vi "FiberWLC_CalcState.vi"(5 "Distribution of states":i32[][](array[numeric]), 7 "Li (bp)":dbl[](array[numeric]), 8 "Gi (kT)":dbl[](array[numeric]), 9 "L handles (bp)":dbl) -> (1 "L free (bp)":dbl[](array[numeric]), 2 "ni*Gi (kT)":dbl[](array[numeric]), 3 "n0":i32[](array[numeric]))   [LabVIEW 2018]
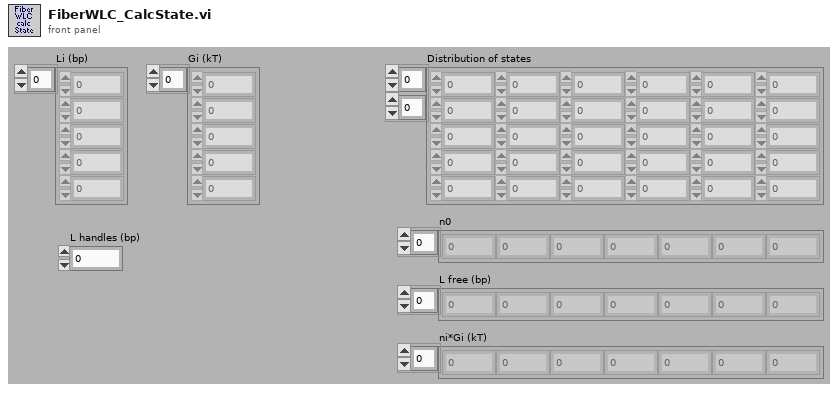
[diagram p1: front panel]
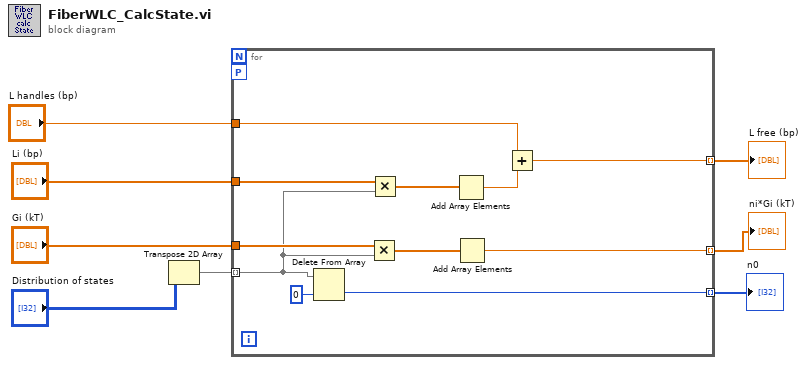
[diagram p0: block diagram]
diagram:
  n1 = Transpose 2D Array(2D array="Distribution of states") -> (transposed array=w7:i32[][])
  n2 = for {
    tunnel: w7 -> [w14] mode=indexing
    tunnel: [w18] -> w5 mode=indexing
    tunnel: "Gi (kT)" -> [w17]
    tunnel: [w16] -> w4 mode=indexing
    tunnel: "Li (bp)" -> [w13]
    tunnel: "L handles (bp)" -> [w10]
    tunnel: [w9] -> w1 mode=indexing
    workers-P: _ -> [_]
    n3 = Delete From Array(array=w14, index=0) -> (deleted portion=w18:i32)  [unwired: 1 in, 1 out]
    n4 = Multiply(x=w17, y=w14) -> (x*y=w15:dbl[])
    n5 = Multiply(x=w13, y=w14) -> (x*y=w12:dbl[])
    n6 = Add Array Elements(numeric array=w12) -> (sum=w11:dbl)
    n7 = Add Array Elements(numeric array=w15) -> (sum=w16:dbl)
    n8 = Add(x=w10, y=w11) -> (x+y=w9:dbl)
  }
  "n0" <- w5
  "ni*Gi (kT)" <- w4
  "L free (bp)" <- w1
